vi "Hova Null setzen.vi"(4 "termination char\n(0xA = '\\n' = LF)  2":u8=3 caption="Endzeichen\n(0xA = '\\n' = LF)" format="%.0x", 6 "Enum":T1, 8 "error in":errorcluster, 9 "VISA resource name out":refnum<visa-resource-name>) -> (0 "error out":errorcluster, 1 "Device":string)   [LabVIEW 2020, in "Linearisierung v2.lvlib" / "Gasteiler.lvlib" / "HovaCal.lvlib"]
uses:
  HovaCal.lvlib
  Aktion_FGV_Kom.ctl
  Aktion_txt.ctl
  Vaporizer.ctl
  <vilib>/Instr/_visa.llb/VISA Configure Serial Port (Instr).vi
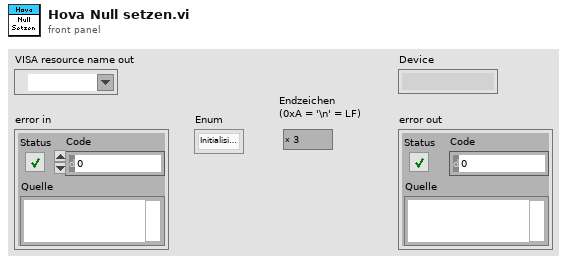
[diagram p1: front panel]
types:
  T1 = typedef "Linearisierung v2.lvlib/Gasteiler.lvlib/HovaCal.lvlib/Aktion_FGV_Kom.ctl" = enum16{"Initialisieren", "Betriebsparameter", "Gase", "Vaporizer", "Dynamische Werte", "Beenden", "Com ändern", "Gase init"}
  T2 = typedef "Linearisierung v2.lvlib/Gasteiler.lvlib/HovaCal.lvlib/Aktion_txt.ctl" = enum16{"ini", "lesen"}
  T3 = enum16{"Lesen", "Vaporizer lesen", "Vaporizer schreiben"}
  T4 = typedef "Linearisierung v2.lvlib/Gasteiler.lvlib/HovaCal.lvlib/Vaporizer.ctl" = cluster{"Pumpe Ein/Aus":dbl, "Wasser / Reagent":dbl, "Reagent dry / wet":dbl, "Reagent":dbl, "min. Temperatur\n160 °C":dbl, "Solltemperatur":dbl, "Wasserkonzentration\nSoll":dbl}
  T5 = cluster{"Pumpe Ein/Aus":bool, "Wasser / Reagent":bool, "Reagent dry / wet":bool, "Reagent":bool, "min. Temperatur\n160 °C":bool, "Solltemperatur":bool, "Wasserkonzentration\nSoll":bool}
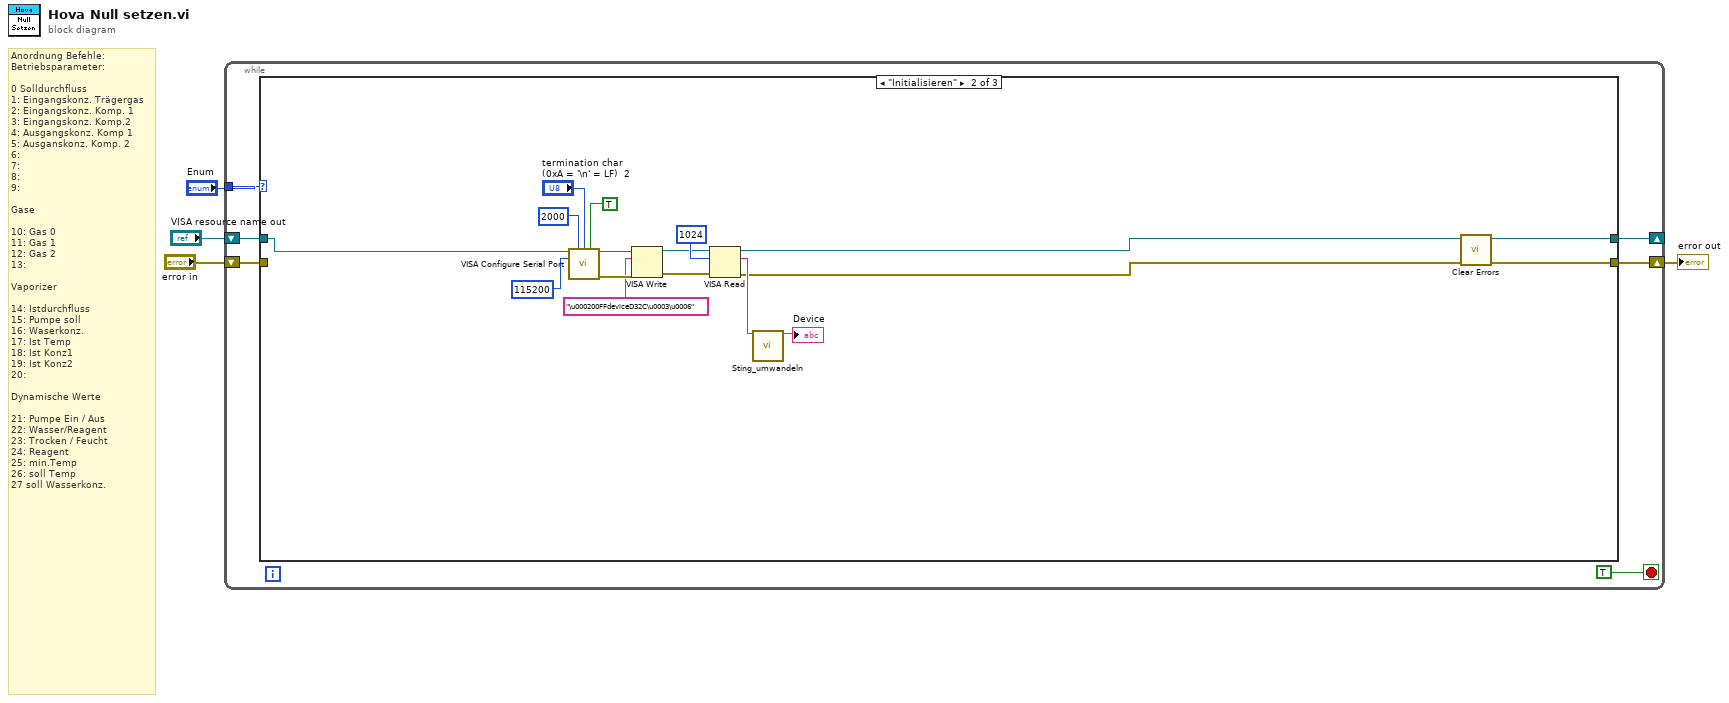
[diagram p0: block diagram]
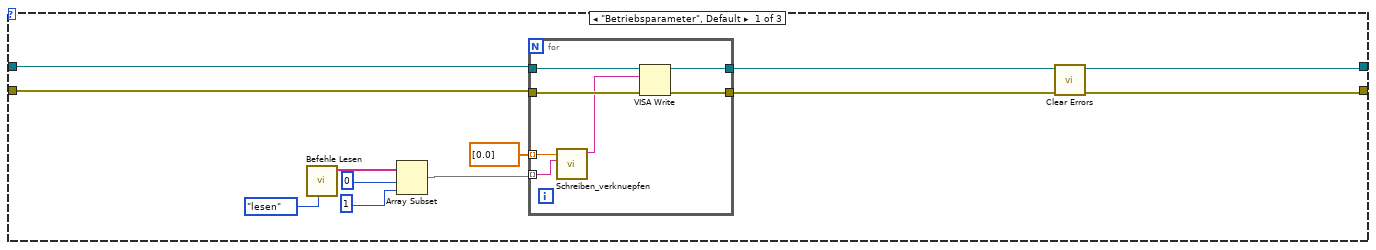
[diagram p2: hidden frame]
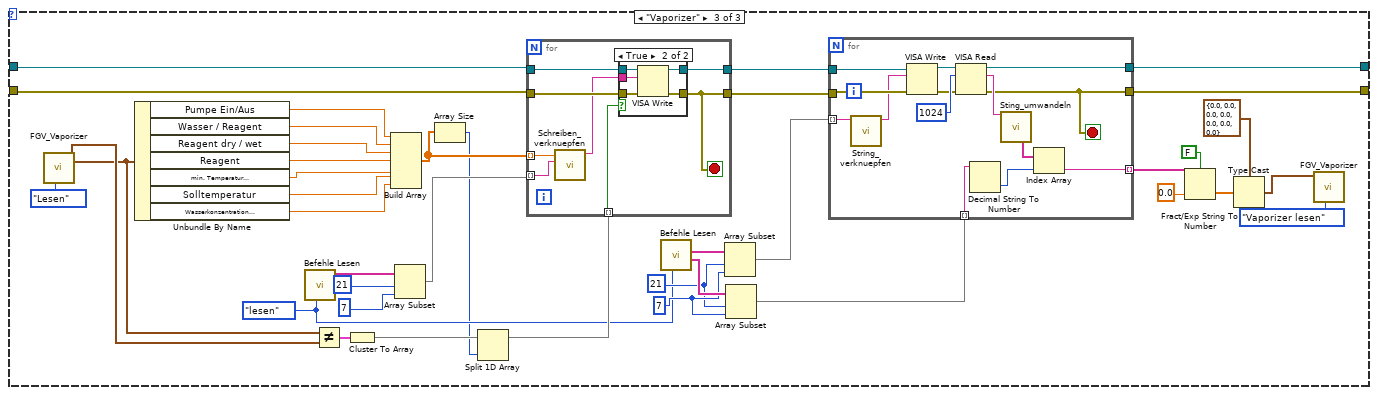
[diagram p3: hidden frame]
diagram:
  # "Anordnung Befehle:\nBetriebsparameter:\n\n0 Solldurchfluss\n1: Eingangskonz. Trägergas\n2: Eingangskonz. Komp. 1\n3: Eingangskonz. Komp.2\n4: Ausgangskonz. Komp 1\n5: Ausganskonz. Komp. 2\n6:\n7:\n8:\n9:\n\nGase\n\n10: Gas 0\n11: Gas 1\n12: Gas 2\n13:\n\nVaporizer\n\n14: Istdurchfluss\n15: Pumpe soll\n16: Waserkonz.\n17: Ist Temp\n18: Ist Konz1\n19: Ist Konz2\n20:\n\nDynamische Werte\n\n21: Pumpe Ein / Aus\n22: Wasser/Reagent\n23: Trocken / Feucht\n24: Reagent\n25: min.Temp\n26: soll Temp\n27 soll Wasserkonz."
  n1 = while {
    tunnel: "Enum" -> [w10]
    shift-right: [w8] -> _
    shift-left: "VISA resource name out" -> [w6]
    shift-right: [w7] -> w4
    shift-left: "error in" -> [w5]
    stop <- TRUE stop-if-true
    n2 = case shown="\"Initialisieren\"" w10 {
      tunnel: [w13 w31 w58] -> w8
      tunnel: [w11 w29 w57] -> w7
      tunnel: w6 -> [w17 w32 w60]
      tunnel: w5 -> [w18 _ w59]
      frame "Betriebsparameter", Default {
        n3 = call "Befehle Lesen.vi"("Enum"=Aktion_txt."lesen") -> ("Schreibbefehl"=w19:string[])  [unwired: 7 in, 3 out]
        n4 = Array Subset(array=w19, index=0 ("Index"), length=1 ("Länge")) -> (w16:string[])
        n5 = for {
          tunnel: w17 -> [w27]
          tunnel: w18 -> [w26]
          tunnel: [w28] -> w13
          tunnel: [w25] -> w12
          tunnel: w16 -> [w23] mode=indexing
          tunnel: dbl[] [0.0] -> [w24] mode=indexing
          n6 = call "Schreiben_verknuepfen.vi"("Order"=w23, "Zahl"=w24) -> ("Verknüpfter String"=w22:string)  [unwired: 8 in, 1 out]
          n7 = VISA Write(VISA resource name=w27, write buffer=w22, error in (no error)=w26) -> (VISA resource name out=w28:refnum<visa-resource-name>, error out=w25:errorcluster)  [unwired: 1 out]
        }
        n8 = call <vilib>:"Clear Errors.vi"("error in (no error)"=w12) -> ("error out"=w11:errorcluster)  [unwired: 5 in, 1 out]
      }
      frame "Initialisieren" {
        n9 = call-poly "VISA Configure Serial Port"("VISA resource name"=w32, "timeout (10sec)"=u32 2000, "termination char\n(0xA = '\\n' = LF)"="termination char\n(0xA = '\\n' = LF)  2", "Enable Termination\nChar (T)"=TRUE ("Enable Termination\nChar (T)"), "baud rate (9600)"=u32 115200) -> ("VISA resource name out"=w37:refnum<visa-resource-name>, "error out"=w38:errorcluster)  [unwired: 9 in]
        n10 = VISA Write(VISA resource name=w37, write buffer="\u000200FFdeviceD32C\u0003\u0006" ("Schreibpuffer"), error in (no error)=w38) -> (VISA resource name out=w34:refnum<visa-resource-name>, error out=w35:errorcluster)  [unwired: 1 out]
        n11 = VISA Read(VISA resource name=w34, byte count=u32 1024 ("Byte-Anzahl"), error in (no error)=w35) -> (VISA resource name out=w31:refnum<visa-resource-name>, read buffer=w39:string, error out=w30:errorcluster)  [unwired: 1 out]
        n12 = call "Sting_umwandeln.vi"("Lesepuffer"=w39) -> ("Device"=→"Device":string)  [unwired: 8 in, 6 out]
        n13 = call <vilib>:"Clear Errors.vi"("error in (no error)"=w30) -> ("error out"=w29:errorcluster)  [unwired: 5 in, 1 out]
      }
      frame "Vaporizer" {
        w63 = Aktion_txt."lesen" ("Enum")
        w73 = 7 ("Index")
        w72 = 21 ("Index")
        n14 = call "FGV_Vaporizer.vi"("Enum"=T3."Lesen") -> ("Vaporizer_schreiben"=w54:T4, "Vaporizer_lesen"=w56:T4)  [unwired: 7 in, 2 out]
        n15 = Unbundle By Name(w54) -> ("Pumpe Ein/Aus"=w53:dbl, "Wasser / Reagent"=w52:dbl, "Reagent dry / wet"=w51:dbl, "Reagent"=w45:dbl, "min. Temperatur\n160 °C"=w50:dbl, "Solltemperatur"=w49:dbl, "Wasserkonzentration\nSoll"=w48:dbl)
        n16 = call "Befehle Lesen.vi"("Enum"=w63) -> ("Schreibbefehl"=w81:string[])  [unwired: 7 in, 3 out]
        n17 = Not Equal?(x=w54, y=w56) -> (x != y?=w65:T5)
        n18 = Cluster To Array(cluster=w65) -> (array=w64:bool[])
        n19 = Build Array(w53, w52, w51, w45, w50, w49, w48) -> (w78:dbl[])
        n20 = Array Subset(array=w81, index=21 ("Index"), length=7 ("Länge")) -> (w79:string[])
        n21 = Array Size(array=w78) -> (size(s)=w62:i32)
        n22 = Split 1D Array(array=w64, index=w62) -> (first subarray=w80:bool[])  [unwired: 1 out]
        n23 = for {
          tunnel: w60 -> [w104]
          tunnel: w59 -> [w103]
          tunnel: [w105] -> w77
          tunnel: [w102] -> w76
          tunnel: w80 -> [w101] mode=indexing
          tunnel: w79 -> [w99] mode=indexing
          tunnel: w78 -> [w100] mode=indexing
          stop <- w102 stop-if-true
          n24 = call "Schreiben_verknuepfen.vi"("Order"=w99, "Zahl"=w100) -> ("Verknüpfter String"=w98:string)  [unwired: 8 in, 1 out]
          n25 = case shown="True" w101 {
            tunnel: [w107 w112] -> w105
            tunnel: w104 -> [w107 w111]
            tunnel: w103 -> [w106 w110]
            tunnel: w98 -> [_ w109]
            tunnel: [w106 w108] -> w102
            frame False {
            }
            frame True {
              n26 = VISA Write(VISA resource name=w111, write buffer=w109, error in (no error)=w110) -> (VISA resource name out=w112:refnum<visa-resource-name>, error out=w108:errorcluster)  [unwired: 1 out]
            }
          }
        }
        n27 = call "Befehle Lesen.vi"("Enum"=w63) -> ("Ausgang für Lesen"=w74:string[], "Lesebefehl"=w75:string[])  [unwired: 7 in, 2 out]
        n28 = Array Subset(array=w75, index=w72, length=w73) -> (w71:string[])
        n29 = Array Subset(array=w74, index=w72, length=w73) -> (w70:string[])
        n30 = for {
          tunnel: w77 -> [w97]
          tunnel: w76 -> [w96]
          tunnel: w71 -> [w87] mode=indexing
          tunnel: [w92] -> w58
          tunnel: [w88] -> w57
          tunnel: w70 -> [w90] mode=indexing
          tunnel: [w89] -> w67 mode=indexing
          stop <- w88 stop-if-true
          n31 = call "String_verknuepfen.vi"("Order"=w87) -> ("Verknüpfter String"=w86:string)  [unwired: 9 in, 1 out]
          n32 = VISA Write(VISA resource name=w97, write buffer=w86, error in (no error)=w96) -> (VISA resource name out=w94:refnum<visa-resource-name>, error out=w93:errorcluster)  [unwired: 1 out]
          n33 = VISA Read(VISA resource name=w94, byte count=u32 1024 ("Byte-Anzahl"), error in (no error)=w93) -> (VISA resource name out=w92:refnum<visa-resource-name>, read buffer=w91:string, error out=w88:errorcluster)  [unwired: 1 out]
          n34 = Decimal String To Number(string=w90) -> (number=w84:i32)  [unwired: 2 in, 1 out]
          n35 = call "Sting_umwandeln.vi"("Lesepuffer"=w91) -> ("Array"=w85:string[])  [unwired: 8 in, 6 out]
          n36 = Index Array(array=w85, index=w84) -> (element=w89:string)
        }
        n37 = Fract/Exp String To Number(use system decimal point (T)=FALSE ("Systemdezimalzeichen verwenden (T)"), string=w67, default (0 dbl)=0.0 ("Standard (0 I32)")) -> (number=w68:dbl[])  [unwired: 1 in, 1 out]
        n38 = Type Cast(type=T4 {"Pumpe Ein/Aus"=0.0, "Wasser / Reagent"=0.0, "Reagent dry / wet"=0.0, "Reagent"=0.0, "min. Temperatur\n160 °C"=0.0, "Solltemperatur"=0.0, "Wasserkonzentration\nSoll"=0.0} ("Vaporizer"), x=w68) -> (*(type *) &x=w46:T4)
        n39 = call "FGV_Vaporizer.vi"("Enum"=T3."Vaporizer lesen", "Vaporizer lesen"=w46) -> ()  [unwired: 6 in, 4 out]
      }
    }
  }
  "error out" <- w4
